vi "Fetch Waveform.vi"(8 "error in (no error)":errorcluster, 10 "Channel":u8, 11 "Base CFG in":refnum<class "Base CFG.lvclass">) -> (0 "error out":errorcluster, 2 "Waveform":waveform(dbl), 3 "Base CFG out":refnum<class "Base CFG.lvclass">)   [LabVIEW 2023, in "CFGs Scope PXI.lvlib" / "Base CFG.lvclass"]
uses:
  Base CFG.lvclass
  Base CFG.lvclass/Base CFG.ctl
  Configuration Base/CFG Base.lvclass
  9a7c277c-3744-422f-a2d5-5dbb7f71351f.vi
  <instrlib>/niScope/Acquire/Fetch/niScope Fetch WDT.vi
  <vilib>/ErrorRing/Error Ring.xnode
  <vilib>/Utility/error.llb/Error Cluster From Error Code.vi
  E:/git/HAL/HAL GOOP4/Configuration Base/CFG Base.lvclass
  E:/git/HAL/HAL GOOP4/Interfaces/IConfigure/IConfigure.lvclass
  E:/git/HAL/HAL GOOP4/Scope/Scope PXI/Base CFG/Base CFG.lvclass
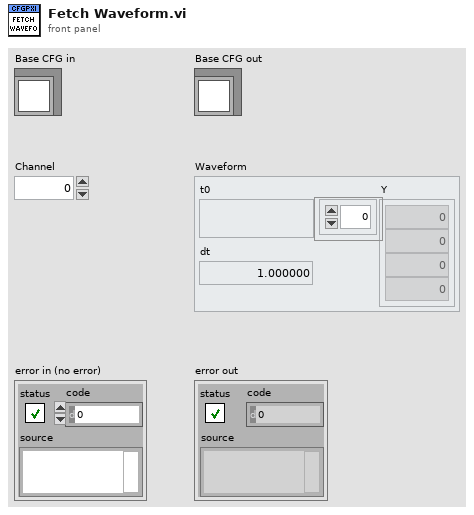
[diagram p1: front panel]
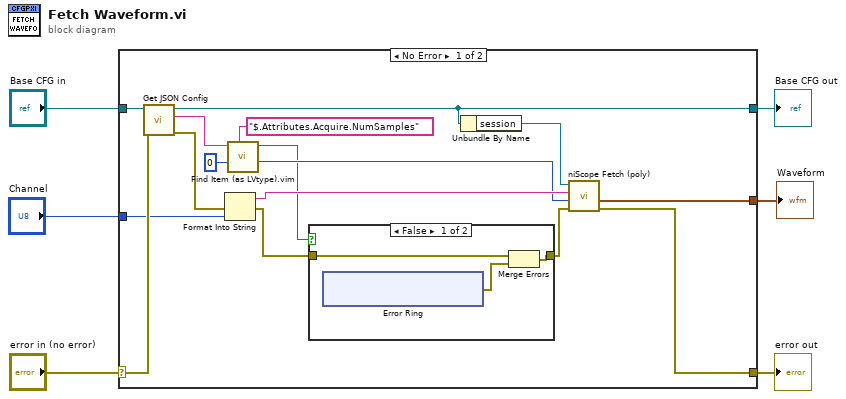
[diagram p0: block diagram]
diagram:
  n1 = case shown="No Error" "error in (no error)" {
    selector: "error in (no error)" -> [w22 w33]
    tunnel: [w21 w33] -> w5
    tunnel: [w12 w32] -> w3
    tunnel: "Base CFG in" -> [w20 w32]
    tunnel: "Channel" -> [w15 _]
    tunnel: [w13 _] -> w1
    frame No Error {
      n2 = call "Get JSON Config.vi"("error in (no error)"=w22, "CFG Base in"=w20) -> ("error out"=w16:errorcluster, "<JSON>Config>"=w17:string, "CFG Base out"=w12:refnum<class "Base CFG.lvclass">)  [unwired: 7 in]
      n3 = Format Into String(error in=w16, w15) -> (resulting string=w14:string, error out=w9:errorcluster)  [unwired: 2 in]
      n4 = call "Find Item (as LVtype).vim"("$Path or Item Name"="$.Attributes.Acquire.NumSamples", "Data Type and Default Value"=0, "JSON"=w17) -> ("Data"=w10:i32, "Found"=w7:bool)  [unwired: 5 in, 2 out]
      n5 = case shown="False" w7 {
        tunnel: w9 -> [w25 w31]
        tunnel: [w24 w31] -> w8
        frame False {
          n6 = xnode "Error Ring"() -> ("error out"=w23:errorcluster)
          n7 = Merge Errors(w25, w23) -> (w24:errorcluster)
        }
        frame True {
        }
      }
      n8 = Unbundle By Name(w12) -> ("session"=w11:refnum<k15>)
      n9 = call-poly <instrlib>:"niScope Fetch (poly).vi"("error in"=w8, "numSamples"=w10, "channels"=w14, "instrument handle"=w11) -> ("error out"=w21:errorcluster, "wfm"=w13:waveform(dbl))  [unwired: 4 in, 2 out]
    }
    frame Error {
    }
  }
  "error out" <- w5
  "Base CFG out" <- w3
  "Waveform" <- w1
